vi "Practica 1 - Entradas y Salidas.vi"() -> ()   [LabVIEW 2023]
panel:
  in  "Controlador de Cadena":string
  out "Indicador Visual":dbl(knob) scale=0.0..10.0
  out "Indicador Perilla":dbl
  out "Indicador de Cadena":string
  out "Indicador boleano":bool
  out "Indicador numerico":dbl
  in  "Controlador Puntero":dbl(slide) scale=0.0..10.0
  in  "Controlador Perilla":dbl(knob) scale=0.0..10.0
  in  "Control Booleano":bool
  in  "Control numerico":dbl
  # "Entradas y salidas"
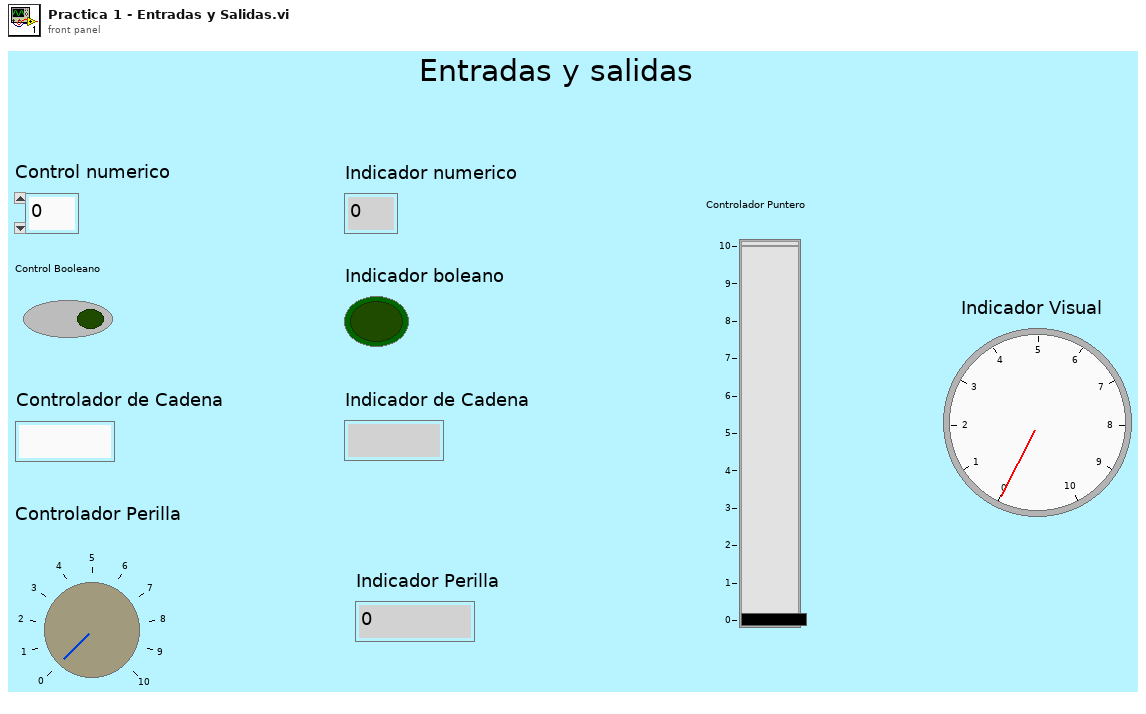
[diagram p1: front panel]
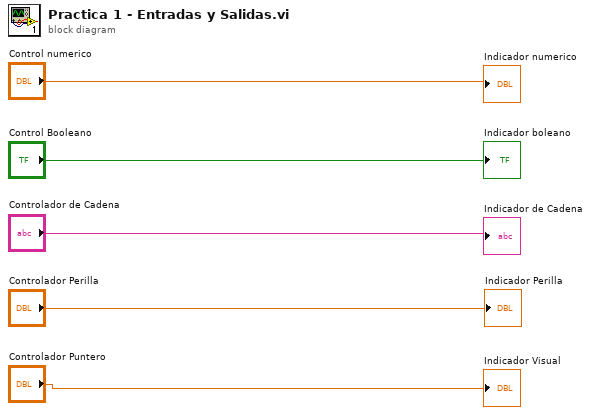
[diagram p0: block diagram]
diagram:
  "Indicador numerico" <- "Control numerico"
  "Indicador boleano" <- "Control Booleano"
  "Indicador de Cadena" <- "Controlador de Cadena"
  "Indicador Perilla" <- "Controlador Perilla"
  "Indicador Visual" <- "Controlador Puntero"
